vi "Open Screenpop.vi"(5 "Screenpop URL Prefix":string, 7 "SR# Cloumn Header":string, 8 "Error In":errorcluster, 9 "Coordinates":cluster{"Horizontal":i32, "Vertical":i32}, 11 "Table Reference":refnum<vi>) -> (0 "Error Out":errorcluster)   [LabVIEW 2017, in "Client.lvlib"]
uses:
  Client.lvlib
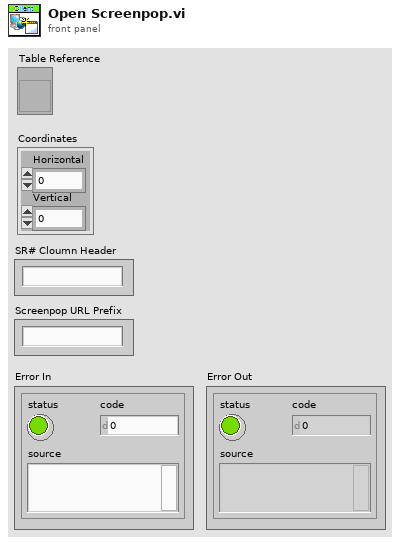
[diagram p1: front panel]
types:
  T1 = typedef "LVRowAndColumnTypeDef.ctl" = cluster{"Row":i32, "Column":i32}
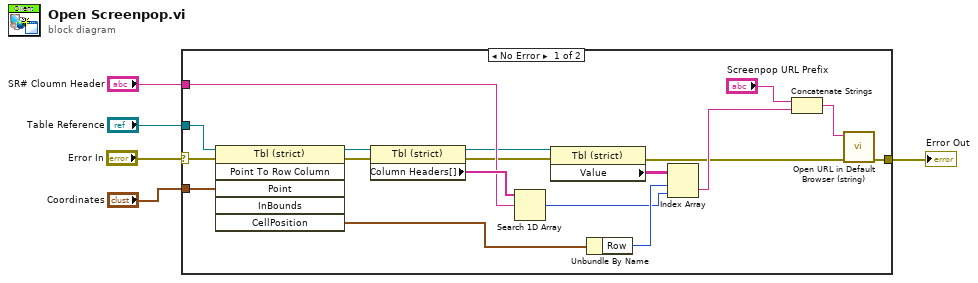
[diagram p0: block diagram]
diagram:
  n1 = case shown="No Error" "Error In" {
    selector: "Error In" -> [w6 w24]
    tunnel: "Coordinates" -> [w22 _]
    tunnel: "Table Reference" -> [w21 _]
    tunnel: "SR# Cloumn Header" -> [w18 _]
    tunnel: [w7 w24] -> w2
    frame No Error {
      n2 = invoke class="Tbl (strict)" method="Point To Row Column"(reference=w21, error in=w6, "Point"=w22) -> (reference out=w20:refnum<vi>, error out=w16:errorcluster, "CellPosition"=w23:T1)  [unwired: 3 in, 3 out]
      n3 = property class="Tbl (strict)"(reference=w20, error in=w16) -> (reference out=w17:refnum<vi>, error out=w15:errorcluster, "Column Headers[]"=w19:string[])
      n4 = Search 1D Array(1D array=w19, element=w18) -> (index of element=w12:i32)  [unwired: 1 in]
      n5 = property class="Tbl (strict)"(reference=w17, error in=w15) -> (error out=w8:errorcluster, "Value"=w14:string[][])  [unwired: 1 out]
      n6 = Unbundle By Name(w23) -> ("Row"=w13:i32)
      n7 = Index Array(array=w14, index (row)=w13, index (col)=w12) -> (element=w10:string)
      n8 = Concatenate Strings("Screenpop URL Prefix", w10) -> (w9:string)
      n9 = call "Open URL in Default Browser (string).vi"("error in (no error)"=w8, "URL"=w9) -> ("error out"=w7:errorcluster)  [unwired: 4 in, 1 out]
    }
    frame Error {
    }
  }
  "Error Out" <- w2
